vi "Load Grid Display.vi"(8 "error in (no error)":errorcluster, 11 "Controller in":refnum<class "Controller.lvclass">) -> (0 "error out":errorcluster, 3 "Controller out":refnum<class "Controller.lvclass">)   [LabVIEW 2024, in "Controller.lvlib" / "Controller.lvclass"]
uses:
  Controller.lvclass
  Applications/National Instruments/LabVIEW 2024 64-bit/vi.lib/ActorFramework/Actor/Actor.lvclass
  MC Screen/MC Screen/Grid Screen.lvclass
  Controller.lvclass/Controller.ctl
  <vilib>/ActorFramework/Actor/Actor.lvclass
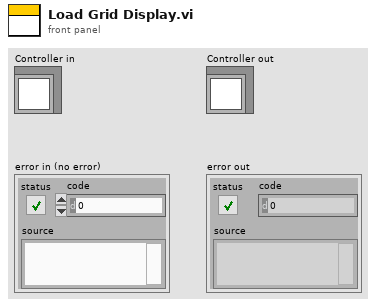
[diagram p1: front panel]
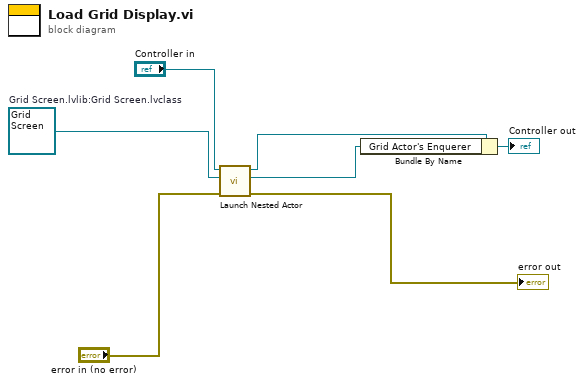
[diagram p0: block diagram]
diagram:
  w5 = refnum<class "Grid Screen.lvclass"> refnum  # Grid Screen.lvlib:Grid Screen.lvclass
  n1 = call <vilib>:"Launch Nested Actor.vi"("error in (no error)"="error in (no error)", "Nested Actor"=w5, "Caller Actor in"="Controller in") -> ("error out"=→"error out":errorcluster, "Nested Actor's Enqueuer"=w2:refnum<class "Message Enqueuer.lvclass">, "Caller Actor out"=w3:refnum<class "Controller.lvclass">)  [unwired: 6 in]
  n2 = Bundle By Name(cluster=w3, "Grid Actor's Enquerer"=w2) -> (→"Controller out":refnum<class "Controller.lvclass">)
